vi "Iteration # to String with Zero Padding.vi"(8 "error in (no error)":errorcluster, 9 "Current #":i32, 11 "Width":u32) -> (0 "error out":errorcluster, 3 "String":string)   [LabVIEW 2017, in "PXImc System Explorer.lvlib"]
uses:
  PXImc System Explorer.lvlib
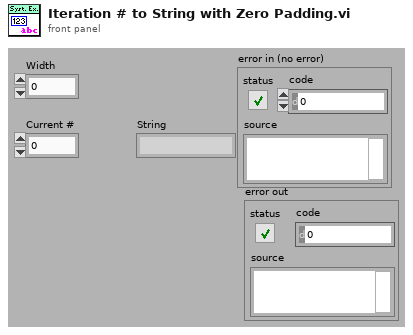
[diagram p1: front panel]
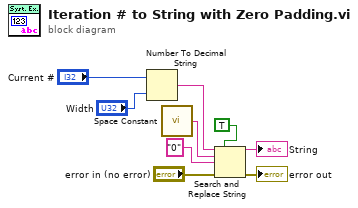
[diagram p0: block diagram]
diagram:
  n1 = Number To Decimal String(number="Current #", width (-)="Width") -> (decimal integer string=w8:string)
  n2 = call <vilib>:"Space Constant.vi"() -> ("String"=w7:string)
  n3 = Search and Replace String(replace all?=TRUE ("replace all? (F)"), input string=w8, search string=w7, replace string="0" ("replace string (\"\")"), error in="error in (no error)") -> (result string=→"String":string, error out=→"error out":errorcluster)  [unwired: 3 in, 2 out]
